vi "Run Turret.vi"(6 "Unwind?":bool, 7 "Search?":bool, 8 "error in (no error)":errorcluster, 9 "Input(deg)":dbl, 10 "Control mode":T1=enum."Offset", 11 "Turret in":refnum<class "Turret.lvclass">) -> (0 "error out":errorcluster, 2 "In Range?":bool, 3 "Turret out":refnum<class "Turret.lvclass">)   [LabVIEW 2019, in "Turret.lvlib" / "Turret.lvclass"]
uses:
  Turret.lvclass
  Controls/Turret control states.ctl
  Turret.lvclass/Turret.ctl
  <vilib>/addons/control/pid/pid.llb/PID (DBL).vi
  <vilib>/addons/control/pid/NI_PID_pid.lvlib
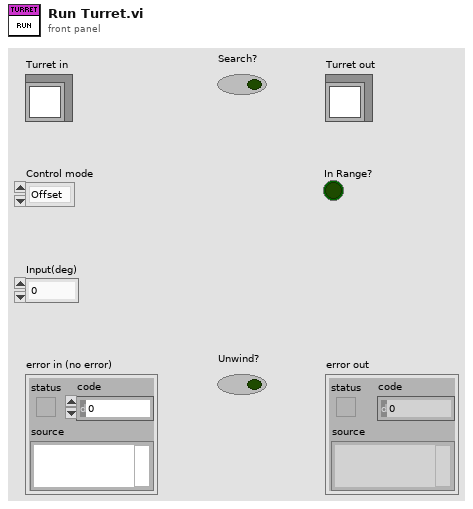
[diagram p1: front panel]
types:
  T1 = typedef "Turret.lvlib/Turret.lvclass/Turret control states.ctl" = enum16{"Position", "Offset", "IMU"}
  T2 = cluster{"proportional gain (Kc)":dbl, "integral time (Ti, min)":dbl, "derivative time (Td, min)":dbl}
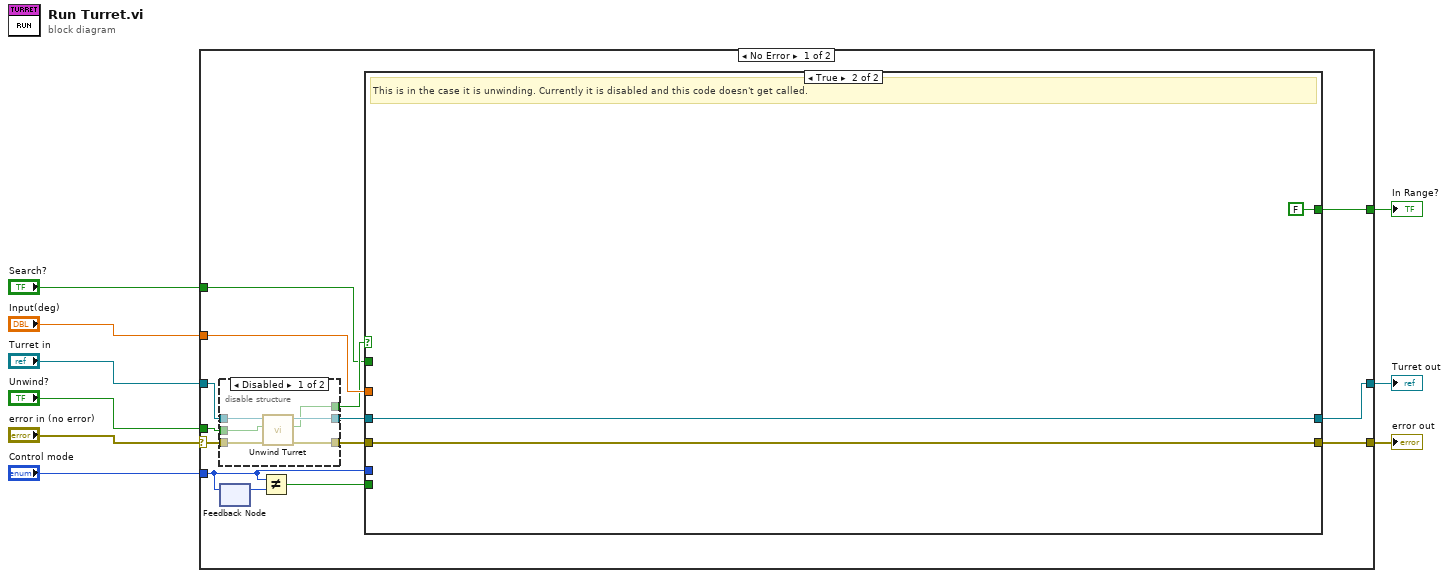
[diagram p0: block diagram]
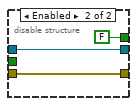
[diagram p2: hidden frame]
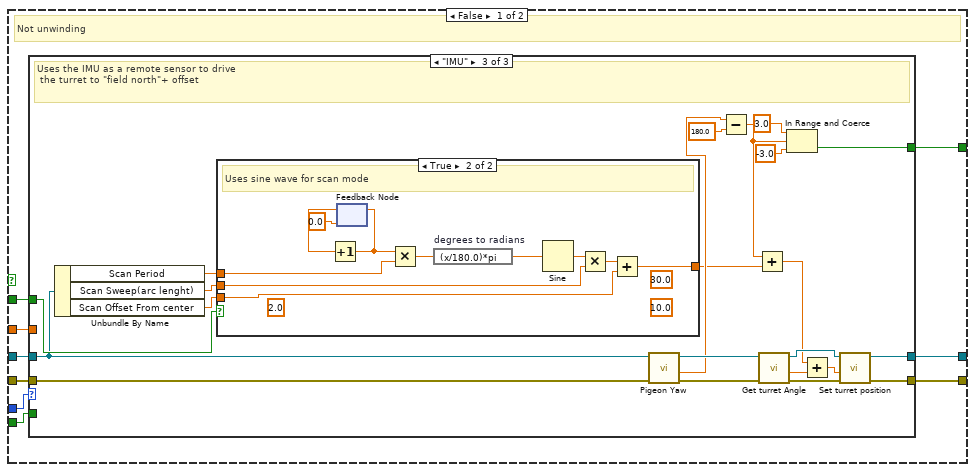
[diagram p3: hidden frame]
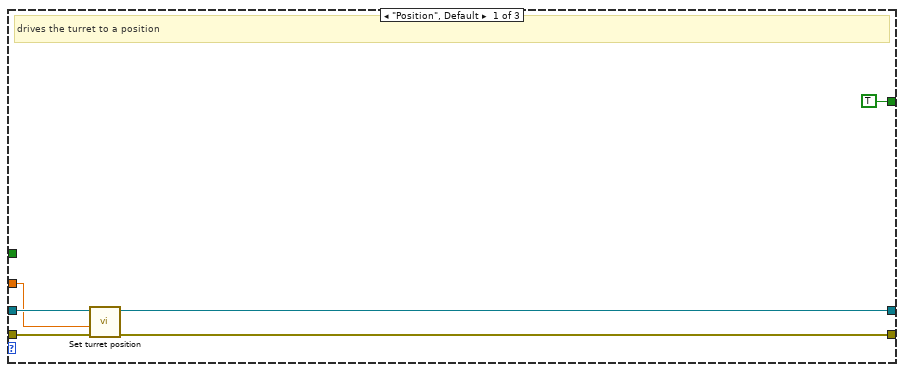
[diagram p4: hidden frame]
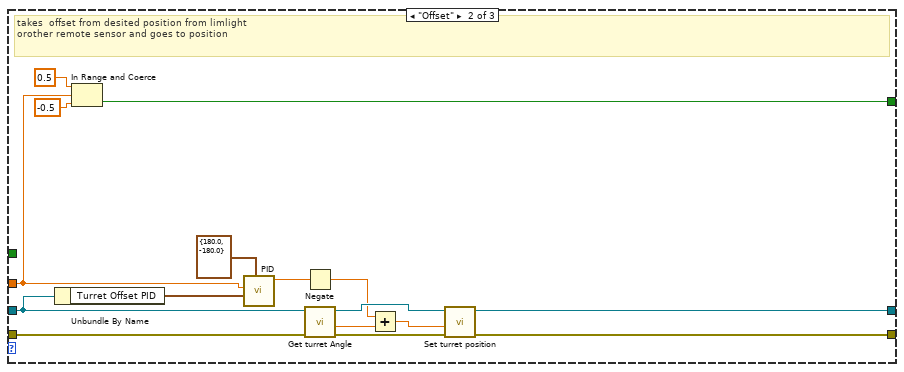
[diagram p5: hidden frame]
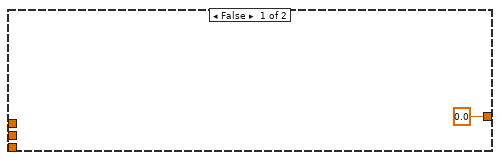
[diagram p6: hidden frame]
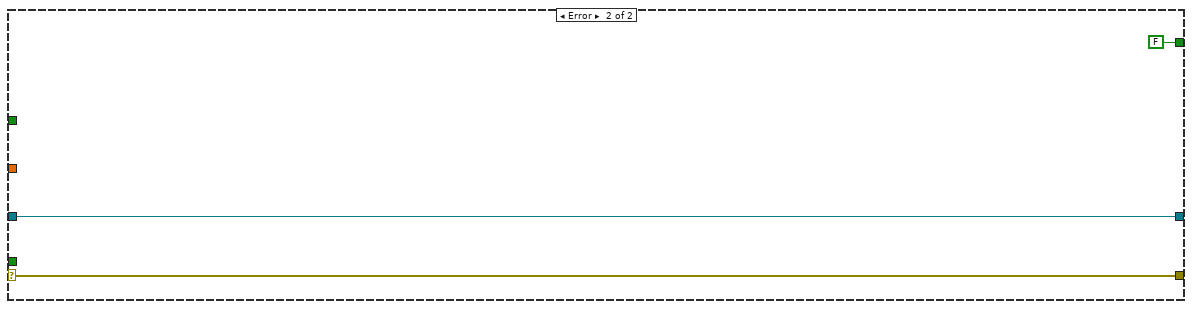
[diagram p7: hidden frame]
diagram:
  n1 = case shown="No Error" "error in (no error)" {
    selector: "error in (no error)" -> [w15 w103]
    tunnel: [w22 w103] -> w8
    tunnel: [w23 w102] -> w6
    tunnel: "Turret in" -> [w17 w102]
    tunnel: "Control mode" -> [w19 _]
    tunnel: "Input(deg)" -> [w18 _]
    tunnel: "Unwind?" -> [w13 _]
    tunnel: "Search?" -> [w11 _]
    tunnel: [w10 FALSE] -> w1
    frame No Error {
      n2 = disable-structure shown="Disabled" {
        disable-tunnel: w17 -> [w29 w32]
        disable-tunnel: [w28 w32] -> w16
        disable-tunnel: w15 -> [w27 w30]
        disable-tunnel: [w26 w30] -> w14
        disable-tunnel: w13 -> [w25 _]
        disable-tunnel: [w24 FALSE] -> w12
        frame Disabled {
          n3 = call "Unwind Turret.vi"("error in (no error)"=w27, "Unwind?"=w25, "Turret in"=w29) -> ("error out"=w26:errorcluster, "Unwinding"=w24:bool, "Turret out"=w28:refnum<class "Turret.lvclass">)  [unwired: 6 in]
        }
        frame Enabled {
        }
      }
      n4 = feedback-in #1(w19) -> ()
      n5 = feedback #1() -> (w21:T1)  [unwired: 1 in]
      n6 = Not Equal?(x=w19, y=w21) -> (x != y?=w20:bool)
      n7 = case shown="True" w12 {
        tunnel: [w41 w99] -> w23
        tunnel: [w40 w100] -> w22
        tunnel: w20 -> [w39 _]
        tunnel: w19 -> [w38 _]
        tunnel: w18 -> [w37 _]
        tunnel: w16 -> [w36 w99]
        tunnel: w14 -> [w35 w100]
        tunnel: w11 -> [w34 _]
        tunnel: [w33 FALSE] -> w10
        frame False {
          # "Not unwinding"
          n8 = case shown="\"IMU\"" w38 {
            tunnel: w37 -> [w45 w51 _]
            tunnel: w36 -> [w47 w53 w72]
            tunnel: [w46 w59 w85] -> w41
            tunnel: w35 -> [w44 w61 w83]
            tunnel: [w43 w60 w84] -> w40
            tunnel: w39 -> [_ _ _]
            tunnel: w34 -> [_ _ w74]
            tunnel: [TRUE w48 w66] -> w33
            frame "Position", Default {
              # "drives the turret to a position"
              n9 = call "Set turret position.vi"("error in (no error)"=w44, "position(deg)"=w45, "Turret in"=w47) -> ("error out"=w43:errorcluster, "Turret out"=w46:refnum<class "Turret.lvclass">)  [unwired: 7 in]
            }
            frame "Offset" {
              # "takes  offset from desited position from limlight \norother remote sensor and goes to position"
              n10 = Unbundle By Name(w53) -> ("Turret Offset PID"=w52:T2)
              n11 = In Range and Coerce(upper limit=0.5, x=w51, lower limit=-0.5) -> (In Range?=w48:bool)  [unwired: 1 out]
              n12 = call-poly <vilib>:"PID.vi"("output range"=cluster{"output high":dbl, "output low":dbl} {"output high"=180.0, "output low"=-180.0}, "PID gains"=w52, "process variable"=w51) -> ("output"=w55:dbl)  [unwired: 7 in, 1 out]
              n13 = Negate(x=w55) -> (-x=w54:dbl)
              n14 = call "Get turret Angle.vi"("error in (no error)"=w61, "Turret in"=w53) -> ("error out"=w63:errorcluster, "Turret Angle(deg)"=w57:dbl, "Turret out"=w62:refnum<class "Turret.lvclass">)  [unwired: 7 in]
              n15 = Add(x=w54, y=w57) -> (x+y=w58:dbl)
              n16 = call "Set turret position.vi"("error in (no error)"=w63, "position(deg)"=w58, "Turret in"=w62) -> ("error out"=w60:errorcluster, "Turret out"=w59:refnum<class "Turret.lvclass">)  [unwired: 7 in]
            }
            frame "IMU" {
              # "Uses the IMU as a remote sensor to drive\n the turret to \"field north\"+ offset"
              n17 = Unbundle By Name(w72) -> ("Scan Period"=w71:dbl, "Scan Sweep(arc lenght)"=w70:dbl, "Scan Offset From center"=w69:dbl)
              n18 = case shown="True" w74 {
                tunnel: [0.0 w90] -> w73
                tunnel: w71 -> [_ w89]
                tunnel: w70 -> [_ w88]
                tunnel: w69 -> [_ w87]
                frame False {
                }
                frame True {
                  (unwired) 10.0
                  (unwired) 30.0
                  (unwired) 2.0 ("y")
                  # "Uses sine wave for scan mode"
                  n19 = feedback #2(0.0) -> (w96:dbl)
                  n20 = Increment(x=w96) -> (x+1=w94:dbl)
                  n21 = feedback-in #2(w94) -> ()
                  n22 = Multiply(x=w94, y=w89) -> (x*y=w97:dbl)
                  n23 = expression code="(x/180.0)*pi" "degrees to radians"(w97) -> (w92:dbl)
                  n24 = Sine(x=w92) -> (sin(x)=w93:dbl)
                  n25 = Multiply(x=w93, y=w88) -> (x*y=w91:dbl)
                  n26 = Add(x=w91, y=w87) -> (x+y=w90:dbl)
                }
              }
              n27 = call "Pigeon Yaw.vi"("error in (no error)"=w83, "Turret in"=w72) -> ("error out"=w80:errorcluster, "Yaw"=w75:dbl, "Turret out"=w81:refnum<class "Turret.lvclass">)  [unwired: 7 in]
              n28 = Subtract(x=w75, y=180.0 ("x")) -> (x-y=w67:dbl)
              n29 = Add(x=w67, y=w73) -> (x+y=w68:dbl)
              n30 = call "Get turret Angle.vi"("error in (no error)"=w80, "Turret in"=w81) -> ("error out"=w79:errorcluster, "Turret Angle(deg)"=w77:dbl, "Turret out"=w78:refnum<class "Turret.lvclass">)  [unwired: 7 in]
              n31 = In Range and Coerce(upper limit=3.0, x=w67, lower limit=-3.0) -> (In Range?=w66:bool)  [unwired: 1 out]
              n32 = Add(x=w68, y=w77) -> (x+y=w76:dbl)
              n33 = call "Set turret position.vi"("error in (no error)"=w79, "position(deg)"=w76, "Turret in"=w78) -> ("error out"=w84:errorcluster, "Turret out"=w85:refnum<class "Turret.lvclass">)  [unwired: 7 in]
            }
          }
        }
        frame True {
          # "This is in the case it is unwinding. Currently it is disabled and this code doesn't get called."
        }
      }
    }
    frame Error {
    }
  }
  "error out" <- w8
  "Turret out" <- w6
  "In Range?" <- w1
